vi "FPGAmain_5782.vi"() -> ()   [LabVIEW 2013]
uses:
  FPGA/DataMode.ctl
  FPGA/Input_5782/5782_states.ctl
  <vilib>/Platform/TimedLoop/XDataNode/timing_clust.ctl
  <vilib>/Platform/TimedLoop/XDataNode/nitl_modes.ctl
  <vilib>/Platform/TimedLoop/XDataNode/wakeup.ctl
  <vilib>/rvi/Emulation/niFpgaSctlEmulationGetInTimedLoop.vi
  <vilib>/rvi/Emulation/niFpgaEmulationReportErrorSimple.vi
  <vilib>/rvi/Emulation/niFpgaGetClockAttributes.vi
  <vilib>/rvi/Emulation/niFpgaCriticalErrorInLSC.vi
  <vilib>/rvi/eio/common/nirviEmuTemplateMethod_errors.vi
  <vilib>/rvi/FIFO/Fifo_Resource/nirvififoEmulationReadFpgaImpl.vi
  <vilib>/rvi/DataTransferAndStorage/Container/Common/niFpgaContainerGetUniqueNameForEmu.vi
  <vilib>/rvi/FIFO/Fifo_Resource/nirvififoEmulationWriteFpgaImpl.vi
  <vilib>/rvi/interface/RandomDataEmulation/nirviRandomDataFPGAFIFO.vi
  <vilib>/rvi/interface/RandomDataEmulation/niFpgaRandomDataHandleErrors.vi
  <vilib>/Platform/TimedLoop/XDataNode/XDataNode.xnode
  <vilib>/eio/EIONode/EIONode.xnode
  <vilib>/rvi/DataTransferAndStorage/Container/XNode/niFpgaContainer.xnode
  <vilib>/rvi/FIFO/Fifo_Resource/nirvififoEmulationRead.vi
  <vilib>/rvi/FIFO/Fifo_Resource/nirvififoEmulationWrite.vi
  <vilib>/rvi/interface/RandomDataEmulation/nirviRandomDataFpgaReadWriteTemplate.vi
  <vilib>/Platform/TimedLoop/XDataNode/XDNodeRunTimeDep.lvlib
  <instrlib>/FlexRIO/Libraries/Helper VIs/NI FlexRIO Helper VIs.lvlib
panel:
  in  "Downsample":fxp<+,8,8>
  in  "enable filter":bool
  in  "new coeffs":bool
  in  "FIR shift":i32
  in  "FIR coeffs":fxp<+/-,18,18>[](array[numeric])
  in  "Set downsample":bool
  in  "CIC Gain":fxp<+/-,32,1>=0.00390625 format="%#_32g"
  in  "trigger samples":i32
  in  "quiet time":i32
  in  "Acquisition running":bool
  in  "Phase output":fxp<+,64,64>[](array[numeric])=[0.0, 0.0, 0.0, 0.0]
  in  "Trigger Acquisition":bool
  in  "5782 record length":i32=128000 caption="Samples Per Trigger" min=1 step=1
  in  "Simulated phase 5782":fxp<+,64,64>[](array[numeric])=[0.0, 0.0]
  in  "Mode":T1
  in  "Phase 5782":fxp<+,64,64>[](array[numeric])=[0.0, 0.0]
  in  "User Command Commit":bool
  in  "User Command":u8
  out "User Command Idle":bool
  out "User Command Status":u8
  in  "User Data 0":u16
  in  "User Data 1":u8
  out "PLL Locked":bool
  out "User Error":bool
  out "Configured?":bool
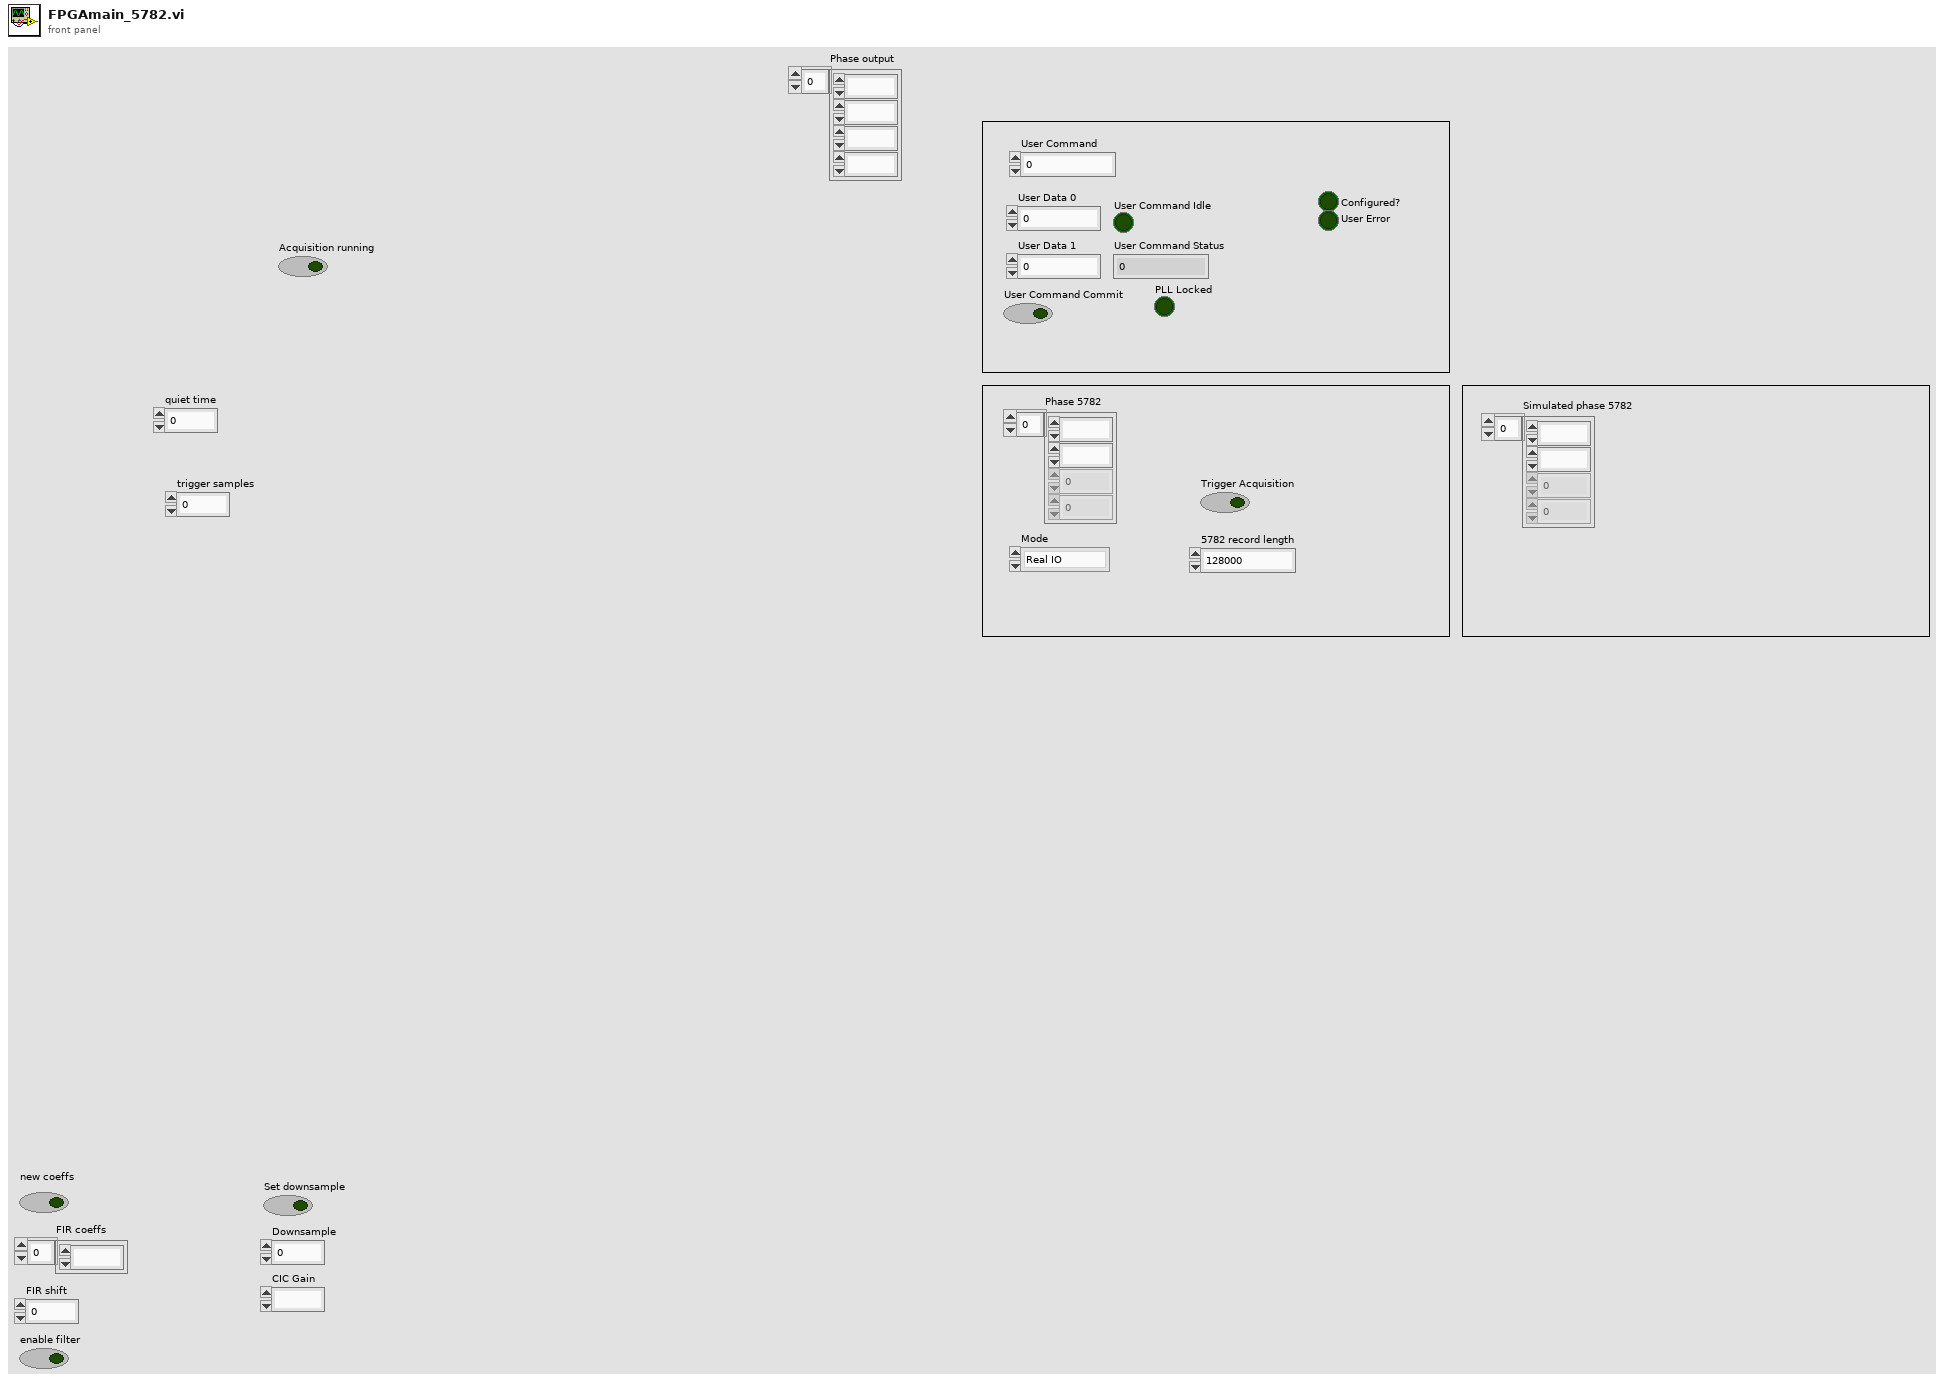
[diagram p1: front panel]
types:
  T1 = typedef "DataMode.ctl" = enum16{"Real IO", "Simulated"}
  T2 = typedef "5782_states.ctl" = enum16{"Wait for trigger", "Acquisition", "Quiet period"}
  T3 = typedef "XDNodeRunTimeDep.lvlib/timing_clust.ctl" = cluster{"Expected End [f-1]":u64, "Actual End [f-1]":u64, "Finished Late? [f-1]":bool, "Expected End [i-1]":u64, "Actual End [i-1]":u64, "Finished Late? [i-1]":bool, "Expected Start [i]":u64, "Actual Start [i]":u64, "Expected Start [f]":u64, "Actual Start [f]":u64, "Source Name":string, "Structure Name":string, "Period":i64, "Deadline":i64, "Offset":i64, "Start":i64, "Priority":i32, "Timeout":i32, "Mode":T4, "Wakeup Reason":T5, "Error":errorcluster, "Source Type":string, "Secondary Source Type":string, "Global End Time":u64, "Global Start Time":u64, "Frame Duration":u64, "Iteration Duration":u64, "Assigned CPU":i32, "I/O Scan Engine Mode":u32}
  T4 = typedef "XDNodeRunTimeDep.lvlib/nitl_modes.ctl" = enum32{"No Change", "Process missed periods, maintain original phase", "Discard missed periods, maintain original phase", "Process missed periods, ignore original phase", "Discard missed periods, ignore original phase"}
  T5 = typedef "XDNodeRunTimeDep.lvlib/wakeup.ctl" = enum32{"Normal", "Aborted", "Asynchronous wakeup", "Timing source error", "Timed loop error", "Timeout"}
  T6 = typedef "I16 array size 2.ctl" = i16[]
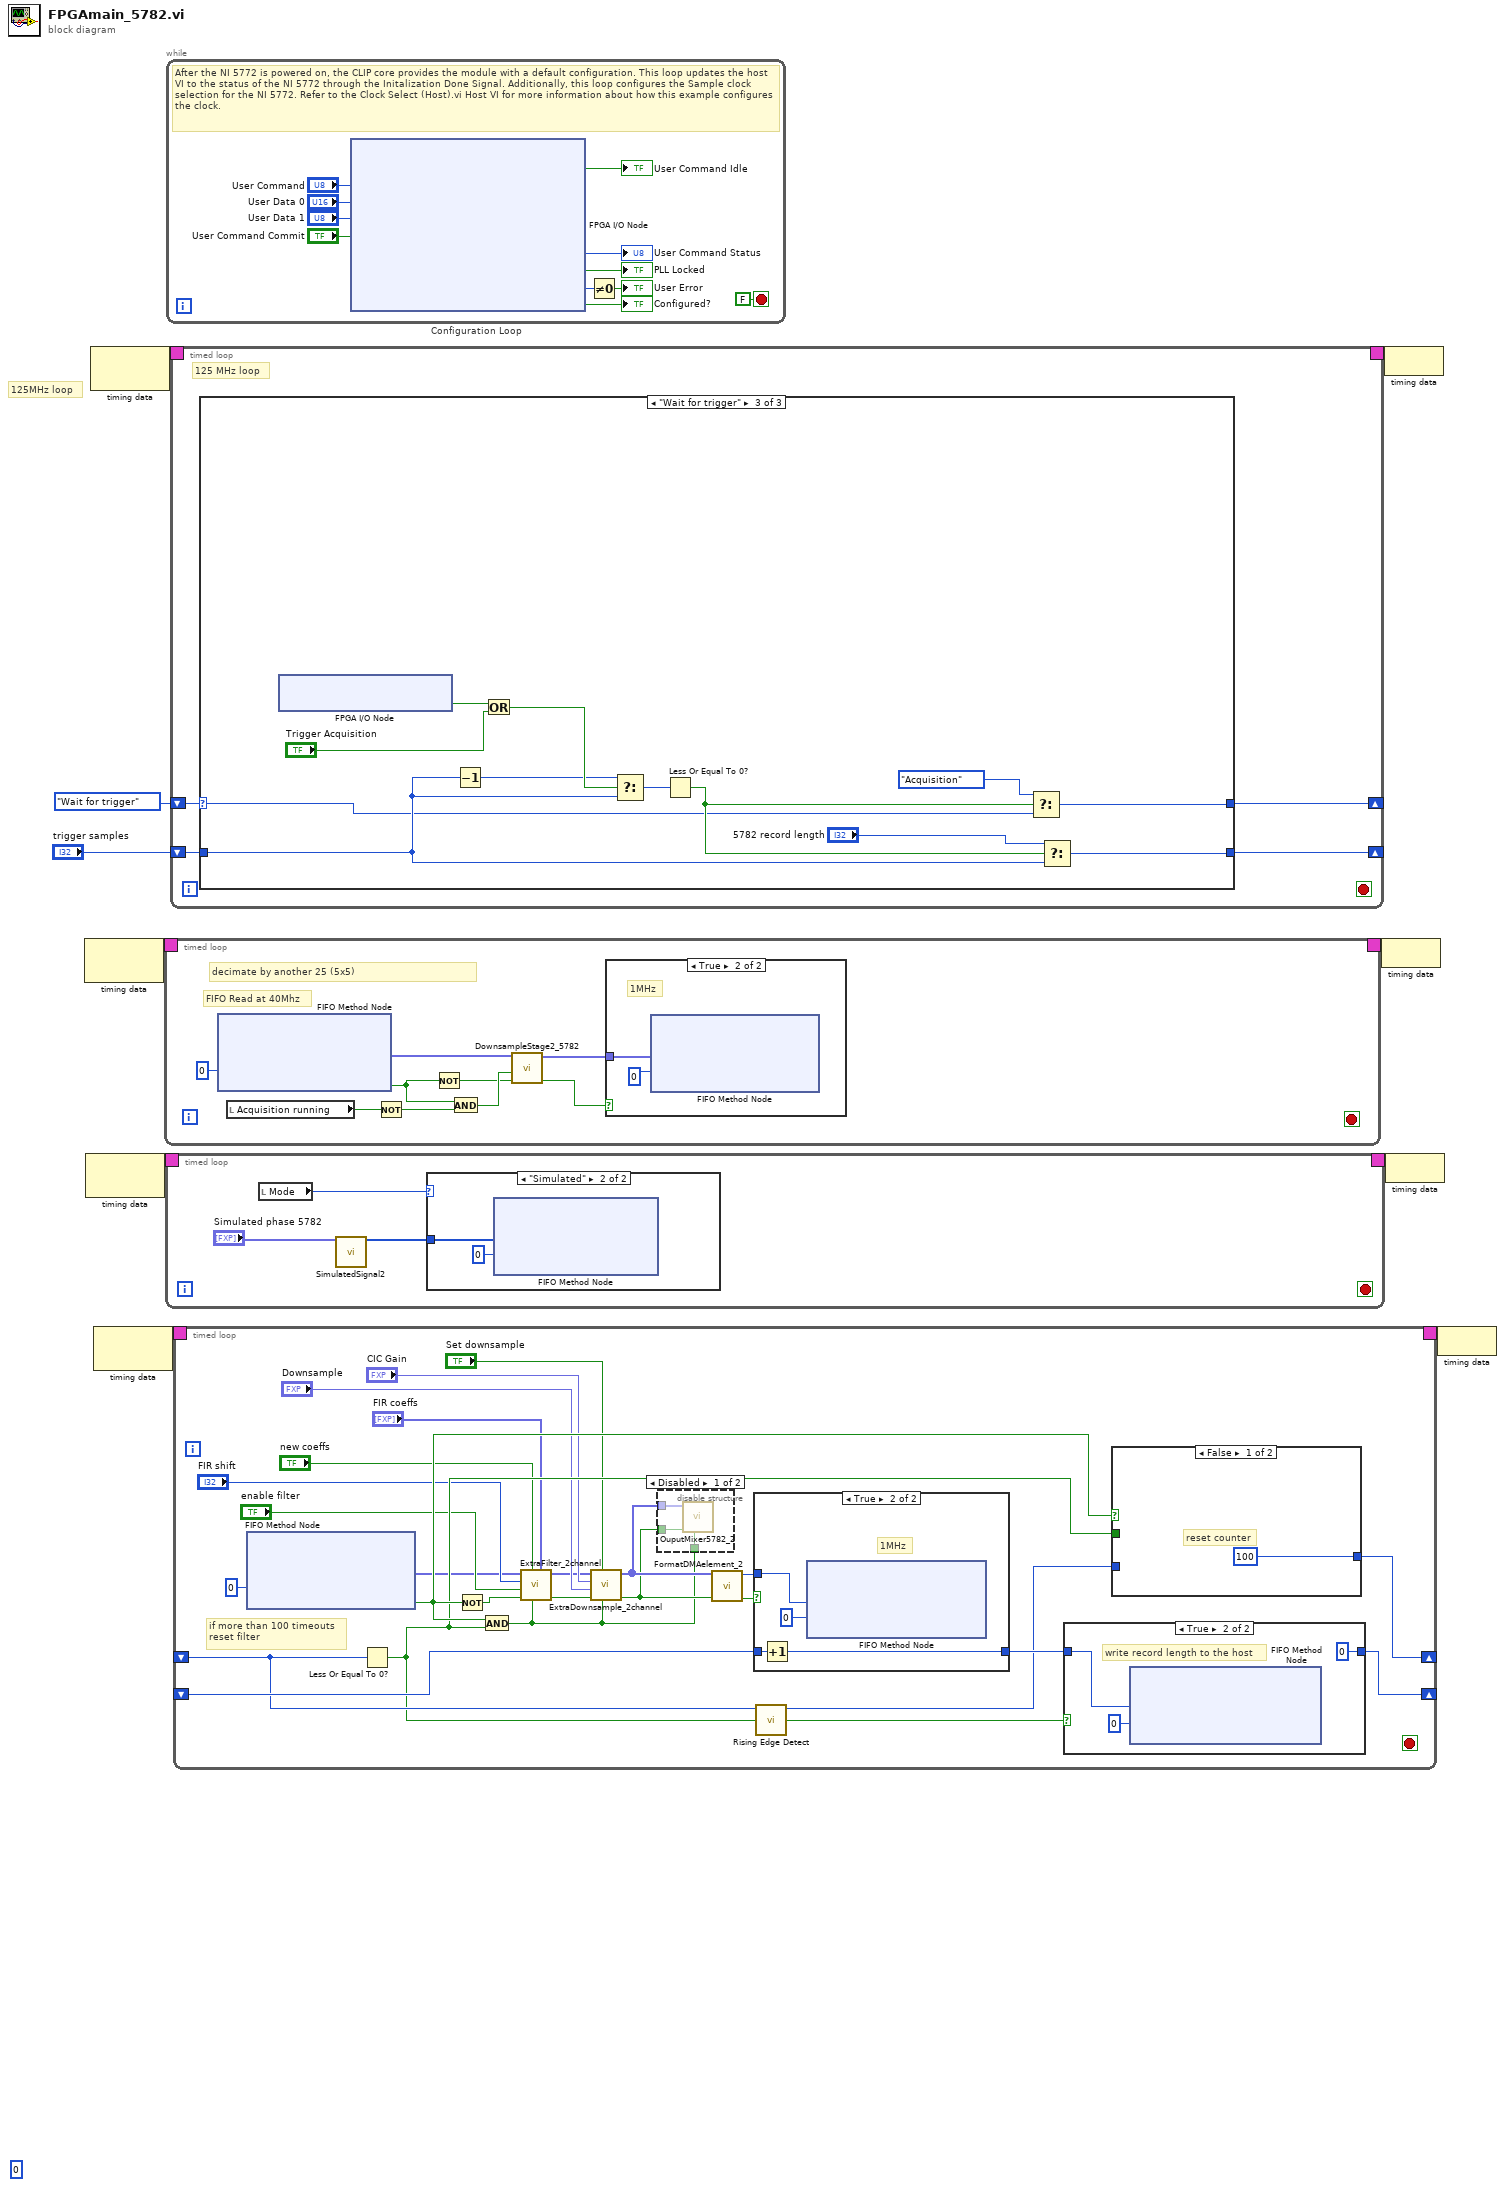
[diagram p0: block diagram]
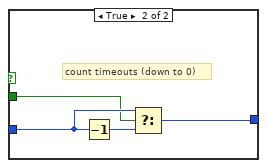
[diagram p3: hidden frame]
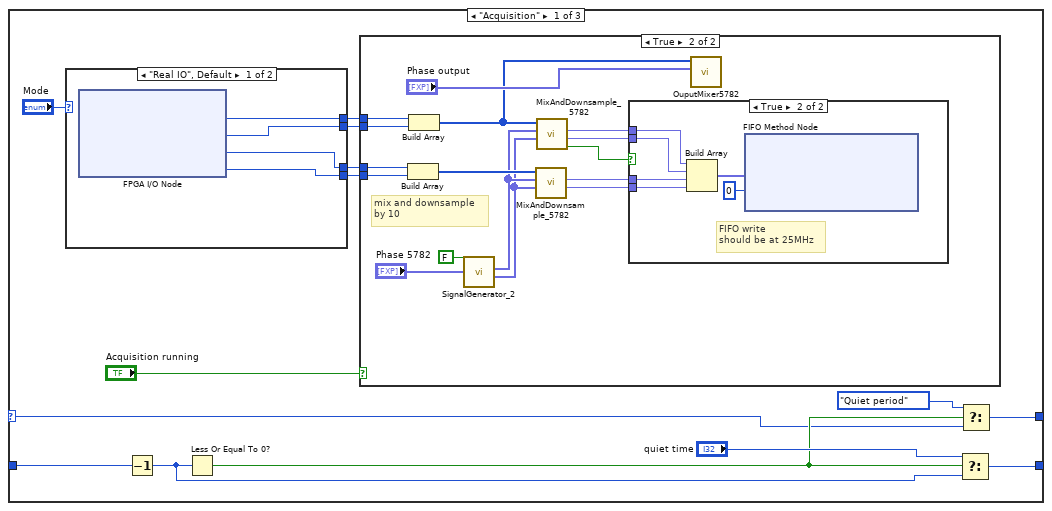
[diagram p6: hidden frame]
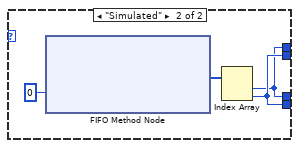
[diagram p9: hidden frame]
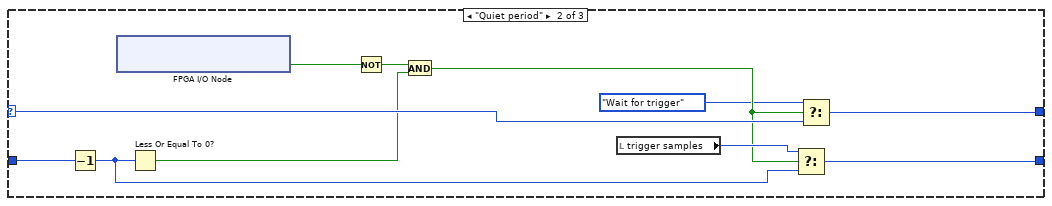
[diagram p10: hidden frame]
diagram:
  (unwired) i16 0
  # "125MHz loop"
  n1 = node-c288() -> (w10:T3)  [unwired: 1 in]
  n2 = node-c288() -> (w8:T3)  [unwired: 1 in]
  n3 = node-c288() -> (w6:T3)  [unwired: 1 in]
  n4 = node-c288() -> (w2:T3)  [unwired: 1 in]
  n5 = timed-loop {
    timing: w10 -> [_]
    timing-out: [_] -> w9
    stop <- _ stop-if-true
    # "FIFO Read at 40Mhz"
    # "decimate by another 25 (5x5)"
    n6 = xnode ("FIFO Method Node")("Timeout"=0) -> ("Element"=w18:fxp<+/-,16,14>[], "Timed Out?"=w13:bool)  [unwired: 1 in, 1 out]
    n7 = local read "Acquisition running"() -> (w15:bool)
    n8 = Not(x=w15) -> (.not. x?=w14:bool)
    n9 = Not(x=w13) -> (.not. x?=w11:bool)
    n10 = And(x=w13, y=w14) -> (x .and. y?=w12:bool)
    n11 = call "DownsampleStage2_5782.vi"("valid in"=w11, "reset"=w12, "Data in"=w18) -> ("valid out"=w16:bool, "data out"=w17:fxp<+/-,16,14>[])  [unwired: 7 in]
    n12 = case shown="True" w16 {
      tunnel: w17 -> [_ w20]
      frame False {
      }
      frame True {
        # "1MHz"
        n13 = xnode ("FIFO Method Node")("Element"=w20, "Timeout"=0) -> ()  [unwired: 1 in, 2 out]
      }
    }
  }
  n14 = timed-loop {
    timing: w8 -> [_]
    timing-out: [_] -> w7
    stop <- _ stop-if-true
    n15 = local read "Mode"() -> (w26:T1)
    n16 = call "SimulatedSignal2.vi"("Phase"="Simulated phase 5782") -> ("output"=w25:T6)  [unwired: 9 in, 1 out]
    n17 = case shown="\"Simulated\"" w26 {
      tunnel: w25 -> [_ w27]
      frame "Real IO", Default {
      }
      frame "Simulated" {
        n18 = xnode ("FIFO Method Node")("Element"=w27, "Timeout"=0) -> ()  [unwired: 1 in, 2 out]
      }
    }
  }
  n19 = while "Configuration Loop" {
    stop <- FALSE stop-if-true
    # "After the NI 5772 is powered on, the CLIP core provides the module with a default configuration. This loop updates the host VI to the status of the NI 5772 through the Initalization Done Signal. Additionally, this loop configures the Sample clock selection for the NI 5772. Refer to the Clock Select (Host).vi Host VI for more information about how this example configures the clock."
    n20 = xnode "FPGA I/O Node"("IO Module\\User Command"="User Command", "IO Module\\User Data 0"="User Data 0", "IO Module\\User Data 1"="User Data 1", "IO Module\\User Command Commit"="User Command Commit") -> ("IO Module\\User Command Idle"=→"User Command Idle":bool, "IO Module\\User Command Status"=→"User Command Status":u8, "IO Module\\PLL Locked"=→"PLL Locked":bool, "IO Module\\User Error"=w36:u8, "IO Module\\Initialization Done"=→"Configured?":bool)  [unwired: 9 in, 9 out]
    n21 = Not Equal To 0?(x=w36) -> (x != 0?=→"User Error":bool)
  }
  n22 = timed-loop {
    timing: w6 -> [_]
    timing-out: [_] -> w5
    shift-right: [w43] -> _
    shift-left: 5782_states."Wait for trigger" ("5782 states") -> [w45]
    shift-right: [w42] -> _
    shift-left: "trigger samples" -> [w44]
    stop <- _ stop-if-true
    # "125 MHz loop"
    n23 = case shown="\"Wait for trigger\"" w45 {
      selector: w45 -> [w54 w96 w106]
      tunnel: w44 -> [w59 w99 w107]
      tunnel: [w53 w95 w105] -> w43
      tunnel: [w56 w98 w104] -> w42
      frame "Acquisition" {
        n24 = case shown="\"Real IO\", Default" "Mode" {
          tunnel: [w85 w86] -> w51
          tunnel: [w84 w87] -> w50
          tunnel: [w83 w86] -> w49
          tunnel: [w82 w87] -> w48
          frame "Real IO", Default {
            n25 = xnode "FPGA I/O Node"() -> ("IO Module\\AI 0 N-1"=w85:i16, "IO Module\\AI 0 N"=w84:i16, "IO Module\\AI 1 N-1"=w83:i16, "IO Module\\AI 1 N"=w82:i16)  [unwired: 4 in, 4 out]
          }
          frame "Simulated" {
            n26 = xnode ("FIFO Method Node")("Timeout"=0) -> ("Element"=w88:i16[])  [unwired: 1 in, 2 out]
            n27 = Index Array(array=w88) -> (element #1=w86:i16, element #2=w87:i16)  [unwired: 2 in]
          }
        }
        n28 = Decrement(x=w59) -> (x-1=w57:i32)
        n29 = Less Or Equal To 0?(x=w57) -> (x <= 0?=w55:bool)
        n30 = case shown="True" "Acquisition running" {
          tunnel: w51 -> [_ w66]
          tunnel: w50 -> [_ w65]
          tunnel: w49 -> [_ w64]
          tunnel: w48 -> [_ w63]
          frame False {
          }
          frame True {
            # "mix and downsample\nby 10"
            n31 = Build Array(w64, w63) -> (w75:i16[])
            n32 = Build Array(w66, w65) -> (w61:i16[])
            n33 = call "SignalGenerator_2.vi"("Phase"="Phase 5782", "reset"=FALSE) -> ("Sine out"=w67:fxp<+/-,16,0>[], "Cosine out"=w68:fxp<+/-,16,0>[])  [unwired: 8 in]
            n34 = call "MixAndDownsample_5782.vi"("Sine in"=w67, "Cosine in"=w68, "Signal Input"=w75) -> ("Q out"=w70:fxp<+/-,16,14>, "I out"=w71:fxp<+/-,16,14>)  [unwired: 6 in, 1 out]
            n35 = call "MixAndDownsample_5782.vi"("Sine in"=w67, "Cosine in"=w68, "Signal Input"=w61) -> ("data valid"=w72:bool, "Q out"=w73:fxp<+/-,16,14>, "I out"=w74:fxp<+/-,16,14>)  [unwired: 6 in]
            n36 = case shown="True" w72 {
              tunnel: w73 -> [_ w81]
              tunnel: w74 -> [_ w78]
              tunnel: w71 -> [_ w77]
              tunnel: w70 -> [_ w76]
              frame False {
              }
              frame True {
                # "FIFO write\nshould be at 25MHz"
                n37 = Build Array(w78, w81, w77, w76) -> (w80:fxp<+/-,16,14>[])
                n38 = xnode ("FIFO Method Node")("Element"=w80, "Timeout"=0) -> ()  [unwired: 1 in, 2 out]
              }
            }
            n39 = call "OuputMixer5782.vi"("Phase output"="Phase output", "Signal Input"=w61) -> ()  [unwired: 10 in]
          }
        }
        n40 = Select(t="quiet time", s=w55, f=w57) -> (s? t:f=w56:i32)
        n41 = Select(t=5782_states."Quiet period" ("5782 states"), s=w55, f=w54) -> (s? t:f=w53:T2)
      }
      frame "Quiet period" {
        n42 = Decrement(x=w99) -> (x-1=w100:i32)
        n43 = xnode "FPGA I/O Node"() -> ("IO Module\\Trigger Input"=w93:bool)  [unwired: 1 in, 1 out]
        n44 = Less Or Equal To 0?(x=w100) -> (x <= 0?=w94:bool)
        n45 = Not(x=w93) -> (.not. x?=w92:bool)
        n46 = And(x=w92, y=w94) -> (x .and. y?=w91:bool)
        n47 = local read "trigger samples"() -> (w97:i32)
        n48 = Select(t=w97, s=w91, f=w100) -> (s? t:f=w98:i32)
        n49 = Select(t=5782_states."Wait for trigger" ("5782 states"), s=w91, f=w96) -> (s? t:f=w95:T2)
      }
      frame "Wait for trigger" {
        n50 = xnode "FPGA I/O Node"() -> ("IO Module\\Trigger Input"=w112:bool)  [unwired: 1 in, 1 out]
        n51 = Decrement(x=w107) -> (x-1=w110:i32)
        n52 = Or(x=w112, y="Trigger Acquisition") -> (x .or. y?=w111:bool)
        n53 = Select(t=w110, s=w111, f=w107) -> (s? t:f=w109:i32)
        n54 = Less Or Equal To 0?(x=w109) -> (x <= 0?=w108:bool)
        n55 = Select(t=5782_states."Acquisition" ("5782 states"), s=w108, f=w106) -> (s? t:f=w105:T2)
        n56 = Select(t="5782 record length", s=w108, f=w107) -> (s? t:f=w104:i32)
      }
    }
  }
  n57 = timed-loop {
    timing: w2 -> [_]
    timing-out: [_] -> w1
    shift-right: [w134] -> _
    shift-left: _ -> [w133]
    shift-right: [w136] -> _
    shift-left: _ -> [w138]
    stop <- _ stop-if-true
    # "if more than 100 timeouts\nreset filter"
    n58 = xnode ("FIFO Method Node")("Timeout"=0) -> ("Element"=w123:fxp<+/-,16,14>[], "Timed Out?"=w135:bool)  [unwired: 1 in, 1 out]
    n59 = Less Or Equal To 0?(x=w133) -> (x <= 0?=w132:bool)
    n60 = Not(x=w135) -> (.not. x?=w121:bool)
    n61 = And(x=w135, y=w132) -> (x .and. y?=w115:bool)
    n62 = call "ExtraFilter_2channel.vi"(5:"new coeffs"="FIR coeffs", "reset"=w115, 7:"new coeffs"="new coeffs", "valid in"=w121, "enable filter"="enable filter", "new shift"="FIR shift", "Data in"=w123) -> ("valid out"=w120:bool, "Data out"=w122:fxp<+/-,16,14>[])  [unwired: 3 in]
    n63 = call "ExtraDownsample_2channel.vi"("reset"=w115, "Set downsample"="Set downsample", "valid in"=w120, "Downsample"="Downsample", "CIC Gain"="CIC Gain", "Data in"=w122) -> ("valid out"=w116:bool, "Data out"=w117:fxp<+/-,16,14>[])  [unwired: 4 in]
    n64 = disable-structure shown="Disabled" {
      disable-tunnel: w117 -> [w142 _]
      disable-tunnel: w116 -> [w141 _]
      disable-tunnel: w115 -> [w140 _]
      frame Disabled {
        n65 = call "OuputMixer5782_2.vi"("reset"=w140, "valid in"=w141, "Data in"=w142) -> ()  [unwired: 8 in, 1 out]
      }
      frame Enabled {
      }
    }
    n66 = call "FormatDMAelement_2.vi"("valid in"=w116, "Data in"=w117) -> ("valid out"=w118:bool, "Element1"=w119:u64)  [unwired: 8 in]
    n67 = case shown="True" w118 {
      tunnel: w119 -> [_ w153]
      tunnel: w138 -> [w152 w155]
      tunnel: [w152 w154] -> w137
      frame False {
      }
      frame True {
        # "1MHz"
        n68 = Increment(x=w155) -> (x+1=w154:i32)
        n69 = xnode ("FIFO Method Node")("Element"=w153, "Timeout"=0) -> ()  [unwired: 1 in, 2 out]
      }
    }
    n70 = call <instrlib>:"Rising Edge Detect.vi"("signal"=w132) -> ("edge detected"=w131:bool)  [unwired: 14 in]
    n71 = case shown="True" w131 {
      tunnel: w137 -> [w148 w149]
      tunnel: [w148 0 ("y")] -> w136
      frame False {
      }
      frame True {
        # "write record length to the host"
        n72 = xnode ("FIFO Method Node")("Element"=w149, "Timeout"=0) -> ()  [unwired: 1 in, 2 out]
      }
    }
    n73 = case shown="False" w135 {
      tunnel: w132 -> [_ w145]
      tunnel: w133 -> [_ w146]
      tunnel: [100 ("y") w144] -> w134
      frame False {
        # "reset counter"
      }
      frame True {
        # "count timeouts (down to 0)"
        n74 = Decrement(x=w146) -> (x-1=w147:i32)
        n75 = Select(t=w146, s=w145, f=w147) -> (s? t:f=w144:i32)
      }
    }
  }
  n76 = node-c288(w9) -> ()
  n77 = node-c288(w5) -> ()
  n78 = node-c288(w7) -> ()
  n79 = node-c288(w1) -> ()
